vi "matrix_h_find.vi"() -> ()   [LabVIEW 2020]
uses:
  <vilib>/userDefined/High Color/IMAQdx.ctl
  <vilib>/Analysis/Matrix/Datatypes/RealMatrix.ctl
  <vilib>/Analysis/7linalg.llb/Solve Linear Equations (multiple right hand).vi
  <vilib>/vision/driver/NI_Vision_Acquisition_Software.lvlib
  <vilib>/Analysis/NI_AALPro.lvlib
  <vilib>/Analysis/Matrix/NI_Matrix.lvlib
panel:
  out "Saving Data 2":bool caption="Saving Data"
  out "output array":T1
  in  "Session In":T2
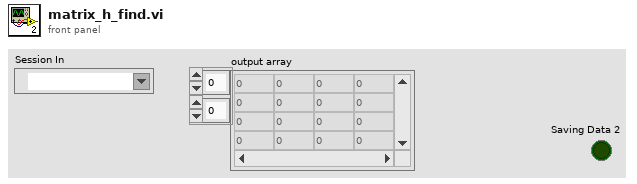
[diagram p1: front panel]
types:
  T1 = typedef "NI_Matrix.lvlib/RealMatrix.ctl" = dbl[][]
  T2 = typedef "IMAQdx.ctl" = refnum<k21>
  T3 = typedef "IMAQ Image.ctl" = refnum<image>
  T4 = typedef "IMAQ Point" = cluster{"X":sgl, "Y":sgl}
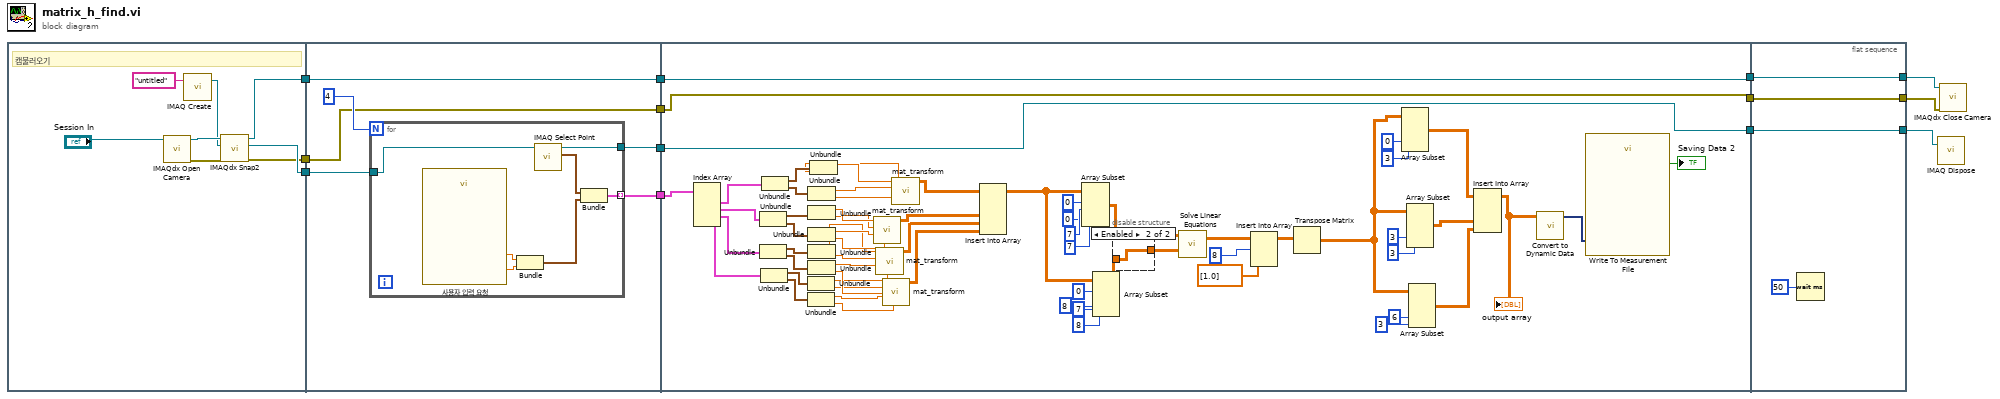
[diagram p0: block diagram]
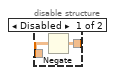
[diagram p2: hidden frame]
diagram:
  n1 = flat-sequence {
    tunnel: [w17] -> w13
    tunnel: [w15] -> w9
    tunnel: [w14] -> w7
    tunnel: w13 -> [w26]
    tunnel: [w25] -> w12
    tunnel: [w24] -> w11
    tunnel: [w23] -> w10
    tunnel: w9 -> [w23]
    tunnel: [w22] -> w8
    tunnel: w7 -> [w22]
    tunnel: w12 -> [w35]
    tunnel: w11 -> [w99]
    tunnel: w10 -> [w37]
    tunnel: w8 -> [w36]
    tunnel: [w37] -> w6
    tunnel: [w36] -> w5
    tunnel: [w35] -> w4
    tunnel: [w104] -> w1
    tunnel: [w105] -> w2
    tunnel: [w106] -> w3
    tunnel: w6 -> [w106]
    tunnel: w5 -> [w105]
    tunnel: w4 -> [w104]
    frame #0 {
      # "캠불러오기"
      n2 = call <vilib>:"IMAQdx Open Camera.vi"("Session In"="Session In") -> ("error out"=w16:errorcluster, "Session Out"=w21:T2)  [unwired: 9 in]
      n3 = call "IMAQ Create"("Image Name"="untitled") -> ("New Image"=w19:T3)  [unwired: 4 in, 1 out]
      n4 = call <vilib>:"IMAQdx Snap2.vi"("error in"=w16, "Image In"=w19, "Session In"=w21) -> ("error out"=w14:errorcluster, "Image Out"=w17:T3, "Session Out"=w15:T2)  [unwired: 6 in]
    }
    frame #1 {
      n5 = for {
        N: 4 -> [_]
        tunnel: w26 -> [w34]
        tunnel: [w29] -> w25
        tunnel: [w28] -> w24 mode=indexing
        n6 = call "사용자 입력 요청"() -> ("v"=w32:dbl, "u"=w33:dbl)  [unwired: 16 in, 2 out]
        n7 = Bundle("u"=w33, "v"=w32) -> (w31:cluster{"u":dbl, "v":dbl})  [unwired: 1 in]
        n8 = call "IMAQ Select Point"("Image In"=w34) -> ("Point"=w30:T4, "Image Out (duplicate)"=w29:T3)  [unwired: 7 in, 2 out]
        n9 = Bundle("Point"=w30, w31) -> (w28:cluster{"Point":T4, cluster{"u":dbl, "v":dbl}})  [unwired: 1 in]
      }
    }
    frame #2 {
      n10 = Index Array(array=w99) -> (element #1=w98:cluster{"Point":T4, cluster{"u":dbl, "v":dbl}}, element #2=w97:cluster{"Point":T4, cluster{"u":dbl, "v":dbl}}, element #3=w96:cluster{"Point":T4, cluster{"u":dbl, "v":dbl}}, element #4=w95:cluster{"Point":T4, cluster{"u":dbl, "v":dbl}})  [unwired: 4 in]
      n11 = Unbundle(w97) -> ("Point"=w92:T4, w91:cluster{"u":dbl, "v":dbl})
      n12 = Unbundle(w96) -> ("Point"=w90:T4, w89:cluster{"u":dbl, "v":dbl})
      n13 = Unbundle(w95) -> ("Point"=w87:T4, w88:cluster{"u":dbl, "v":dbl})
      n14 = Unbundle(w98) -> ("Point"=w94:T4, w93:cluster{"u":dbl, "v":dbl})
      n15 = Unbundle(w87) -> ("X"=w74:sgl, "Y"=w73:sgl)
      n16 = Unbundle(w88) -> ("u"=w72:dbl, "v"=w71:dbl)
      n17 = Unbundle(w93) -> ("u"=w84:dbl, "v"=w83:dbl)
      n18 = Unbundle(w92) -> ("X"=w82:sgl, "Y"=w81:sgl)
      n19 = Unbundle(w91) -> ("u"=w79:dbl, "v"=w80:dbl)
      n20 = Unbundle(w90) -> ("X"=w78:sgl, "Y"=w77:sgl)
      n21 = Unbundle(w89) -> ("u"=w76:dbl, "v"=w75:dbl)
      n22 = Unbundle(w94) -> ("X"=w86:sgl, "Y"=w85:sgl)
      n23 = call "mat_transform.vi"("v"=w80, "u"=w79, "Y"=w81, "X"=w82) -> ("Real Matrix"=w69:T1)  [unwired: 7 in]
      n24 = call "mat_transform.vi"("v"=w75, "u"=w76, "Y"=w77, "X"=w78) -> ("Real Matrix"=w68:T1)  [unwired: 7 in]
      n25 = call "mat_transform.vi"("v"=w71, "u"=w72, "Y"=w73, "X"=w74) -> ("Real Matrix"=w67:T1)  [unwired: 7 in]
      n26 = call "mat_transform.vi"("v"=w83, "u"=w84, "Y"=w85, "X"=w86) -> ("Real Matrix"=w70:T1)  [unwired: 7 in]
      n27 = Insert Into Array(array=w70, new element #1=w69, new element #2=w68, new element #3=w67) -> (w62:T1)  [unwired: 2 in]
      n28 = Array Subset(array=w62, index (row)=0 ("row 1"), length (row)=7 ("row N"), index (col)=0 ("column 1"), length (col)=7 ("column N")) -> (w55:T1)
      n29 = Array Subset(array=w62, index (row)=0 ("row 1"), length (row)=7 ("row N"), index (col)=8 ("column 1"), length (col)=8 ("column N")) -> (w57:T1)
      n30 = disable-structure shown="Enabled" {
        disable-tunnel: w57 -> [w101 w102]
        disable-tunnel: [w100 w102] -> w56
        frame Disabled {
          n31 = Negate(x=w101) -> (-x=w100:T1)
        }
        frame Enabled {
        }
      }
      n32 = call-poly <vilib>:"Solve Linear Equations.vi"("Known Matrix"=w56, "Input Matrix"=w55) -> ("Solution Matrix"=w53:T1)  [unwired: 1 in, 1 out]
      n33 = Insert Into Array(array=w53, index (row)=8 ("index"), new element=dbl[] [1.0] ("new element/subarray")) -> (w51:T1)  [unwired: 1 in]
      n34 = Transpose Matrix(1:w51) -> (0:w50:T1)
      n35 = Array Subset(array=w50, index (col)=0 ("index"), length (col)=3 ("length")) -> (w43:T1)  [unwired: 2 in]
      n36 = Array Subset(array=w50, index (col)=3 ("index"), length (col)=3 ("length")) -> (w42:T1)  [unwired: 2 in]
      n37 = Array Subset(array=w50, index (col)=6 ("index"), length (col)=3 ("length")) -> (w41:T1)  [unwired: 2 in]
      n38 = Insert Into Array(array=w43, new element #1=w42, new element #2=w41) -> (w40:T1)  [unwired: 2 in]
      "output array" <- w40
      n39 = call "Convert to Dynamic Data"("2D Array"=w40) -> ("Dynamic Data Type"=w39:dynamicdata)  [unwired: 3 in]
      n40 = call "Write To Measurement File"("Signals"=w39) -> ("Saving Data"=→"Saving Data 2":bool)  [unwired: 16 in, 2 out]
    }
    frame #3 {
      n41 = Wait (ms)(milliseconds to wait=u32 50) -> ()  [unwired: 1 out]
    }
  }
  n42 = call "IMAQ Dispose"("Image"=w1) -> ()  [unwired: 5 in, 1 out]
  n43 = call <vilib>:"IMAQdx Close Camera.vi"("error in"=w2, "Session In"=w3) -> ()  [unwired: 9 in, 1 out]
